vi "Read gTargTime.vi"(8 "error in (no error)":errorcluster, 11 "GWTargetPositionParameters in":refnum<class "GWTargetPositionParameters.lvclass">) -> (0 "error out":errorcluster, 2 "gTargTime":timestamp, 3 "GWTargetPositionParameters out":refnum<class "GWTargetPositionParameters.lvclass">)   [LabVIEW 2014, in "TCSDataDefinitions.lvlib" / "TCSGuiderStatus.lvlib" / "GWTargetPositionParameters.lvclass"]
uses:
  GWTargetPositionParameters.lvclass
  GWTargetPositionParameters.lvclass/GWTargetPositionParameters.ctl
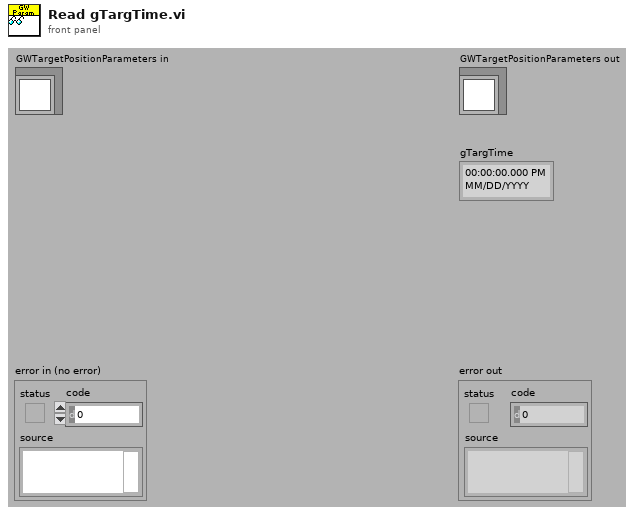
[diagram p1: front panel]
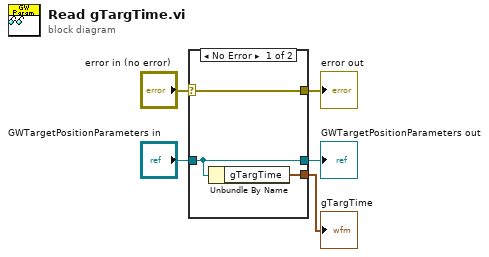
[diagram p0: block diagram]
diagram:
  n1 = case shown="No Error" "error in (no error)" {
    selector: "error in (no error)" -> [w8 w9]
    tunnel: [w8 w9] -> w4
    tunnel: [w7 w10] -> w2
    tunnel: "GWTargetPositionParameters in" -> [w7 w10]
    tunnel: [w6 _] -> w1
    frame No Error {
      n2 = Unbundle By Name(w7) -> ("gTargTime"=w6:timestamp)
    }
    frame Error {
    }
  }
  "error out" <- w4
  "GWTargetPositionParameters out" <- w2
  "gTargTime" <- w1
